vi "translateMotorStatus.vi"(0 "Controller in":refnum<class "_Controller.lvclass">, 2 "actual value":u32, 5 "error in (no error)":errorcluster) -> (14 "Controller out":refnum<class "_Controller.lvclass">, 16 "motion_state":T1=enum."CONST", 17 "other_states (for use in overiding classes)":T1[](array[typedef]), 19 "error out":errorcluster)   [LabVIEW 2013, in "classes.lvlib" / "_Controller.lvclass"]
doc: "Retrieves the Controller's current state\n\nProduced By:\n\n<B>Kod Integrations, LLC</B>\n4835 Marianne Drive\nMount Airy, MD 21771\nhttp://www.kodintegrations.com\nemail: info@kodintegrations.com\nphone: (240) 687-1288"
uses:
  _Controller.lvclass
  common/controls/motor_status.ctl
  libraries/common.lvlib
panel:
  out "other state (for use in overiding classes)":bool[](array[boolean])
  out "motion state":bool[](array[boolean])
  out "actual bits":bool[](array[boolean])
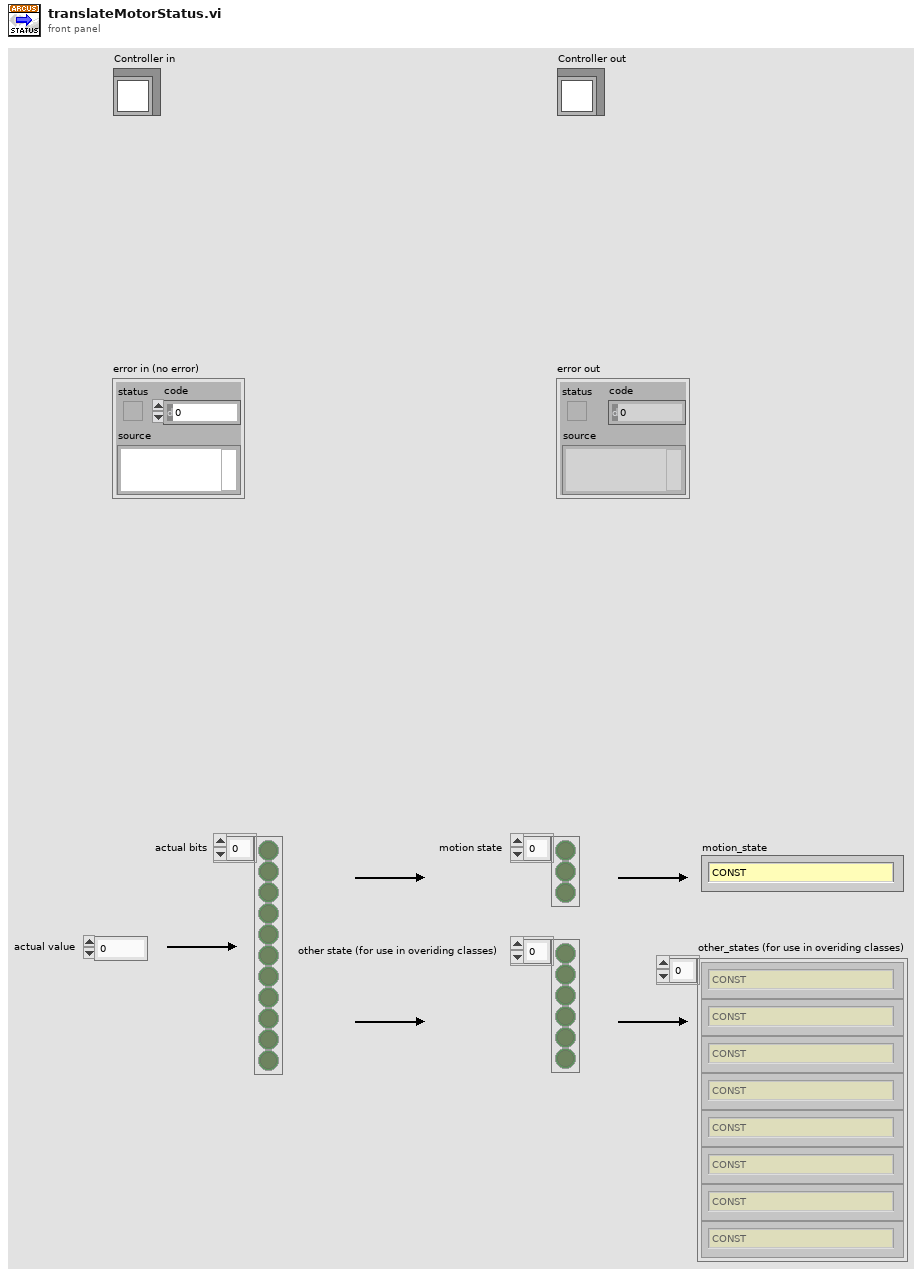
[diagram p1: front panel]
types:
  T1 = typedef "common.lvlib/motor_status.ctl" = enum16{"IDLE", "CONST", "ACCEL", "DECEL", "HOME_SWITCH", "-LIMIT_SWITCH", "+LIMIT_SWITCH", "-LIMIT_ERR", "+LIMIT_ERR", "COMM_TIMEOUT", "ALARM_INPUT", "ALARM_ERROR", "TOC_TIMEOUT_STATUS", "LATCH_INPUT_STATUS", "Z_INDEX_STATUS"}
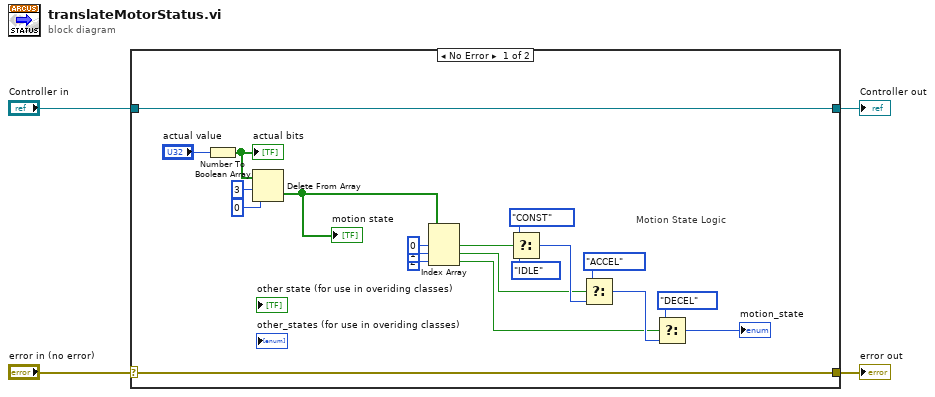
[diagram p0: block diagram]
diagram:
  n1 = case shown="No Error" "error in (no error)" {
    selector: "error in (no error)" -> [w23 w26]
    tunnel: [w23 w26] -> w3
    tunnel: [w24 w25] -> w1
    tunnel: "Controller in" -> [w24 w25]
    frame No Error {
      # "Motion State Logic"
      n2 = Number To Boolean Array(number="actual value") -> (Boolean array=w6:bool[])
      "actual bits" <- w6
      n3 = Delete From Array(array=w6, length=3, index=0) -> (deleted portion=w22:bool[])  [unwired: 1 out]
      "motion state" <- w22
      n4 = Index Array(array=w22, index #1=0 ("index"), index #2=1 ("index"), index #3=2 ("index")) -> (element #1=w13:bool, element #2=w15:bool, element #3=w19:bool)
      n5 = Select(t=motor_status."CONST" ("motion_state"), s=w13, f=motor_status."IDLE" ("motion_state")) -> (s? t:f=w16:T1)
      n6 = Select(t=motor_status."ACCEL" ("motion_state"), s=w15, f=w16) -> (s? t:f=w20:T1)
      n7 = Select(t=motor_status."DECEL" ("motion_state"), s=w19, f=w20) -> (s? t:f=→"motion_state":T1)
    }
    frame Error {
    }
  }
  "error out" <- w3
  "Controller out" <- w1
